vi "Telop Counter Variable.vi"() -> ()   [LabVIEW 2017]
panel:
  in  "Counter":dbl
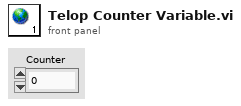
[diagram p1: front panel]
diagram:
